vi "fifoTesting.vi"   [LabVIEW 2016]
uses:
  <vilib>/Platform/TimedLoop/XDataNode/timing_clust.ctl
  <vilib>/Platform/TimedLoop/XDataNode/nitl_modes.ctl
  <vilib>/Platform/TimedLoop/XDataNode/wakeup.ctl
  <vilib>/rvi/Emulation/niFpgaSctlEmulationGetInTimedLoop.vi
  <vilib>/rvi/Emulation/niFpgaEmulationReportErrorSimple.vi
  <vilib>/rvi/Emulation/niFpgaGetClockAttributes.vi
  <vilib>/rvi/Emulation/niFpgaCriticalErrorInLSC.vi
  <vilib>/rvi/interface/RandomDataEmulation/niFpgaRandomDataHandleErrors.vi
  <vilib>/platform/TimedLoop/XDataNode/XDataNode.xnode
  <vilib>/rvi/DataTransferAndStorage/Container/XNode/niFpgaContainer.xnode
  <vilib>/rvi/interface/RandomDataEmulation/nirviRandomDataFpgaReadWriteTemplate.vi
  <vilib>/Platform/TimedLoop/XDataNode/XDNodeRunTimeDep.lvlib
types:
  T1 = typedef "XDNodeRunTimeDep.lvlib/timing_clust.ctl" = cluster{"Expected End [f-1]":u64, "Actual End [f-1]":u64, "Finished Late? [f-1]":bool, "Expected End [i-1]":u64, "Actual End [i-1]":u64, "Finished Late? [i-1]":bool, "Expected Start [i]":u64, "Actual Start [i]":u64, "Expected Start [f]":u64, "Actual Start [f]":u64, "Source Name":string, "Structure Name":string, "Period":i64, "Deadline":i64, "Offset":i64, "Start":i64, "Priority":i32, "Timeout":i32, "Mode":T2, "Wakeup Reason":T3, "Error":errorcluster, "Source Type":string, "Secondary Source Type":string, "Global End Time":u64, "Global Start Time":u64, "Frame Duration":u64, "Iteration Duration":u64, "Assigned CPU":i32, "I/O Scan Engine Mode":u32}
  T2 = typedef "XDNodeRunTimeDep.lvlib/nitl_modes.ctl" = enum32{"No Change", "Process missed periods, maintain original phase", "Discard missed periods, maintain original phase", "Process missed periods, ignore original phase", "Discard missed periods, ignore original phase"}
  T3 = typedef "XDNodeRunTimeDep.lvlib/wakeup.ctl" = enum32{"Normal", "Aborted", "Asynchronous wakeup", "Timing source error", "Timed loop error", "Timeout"}
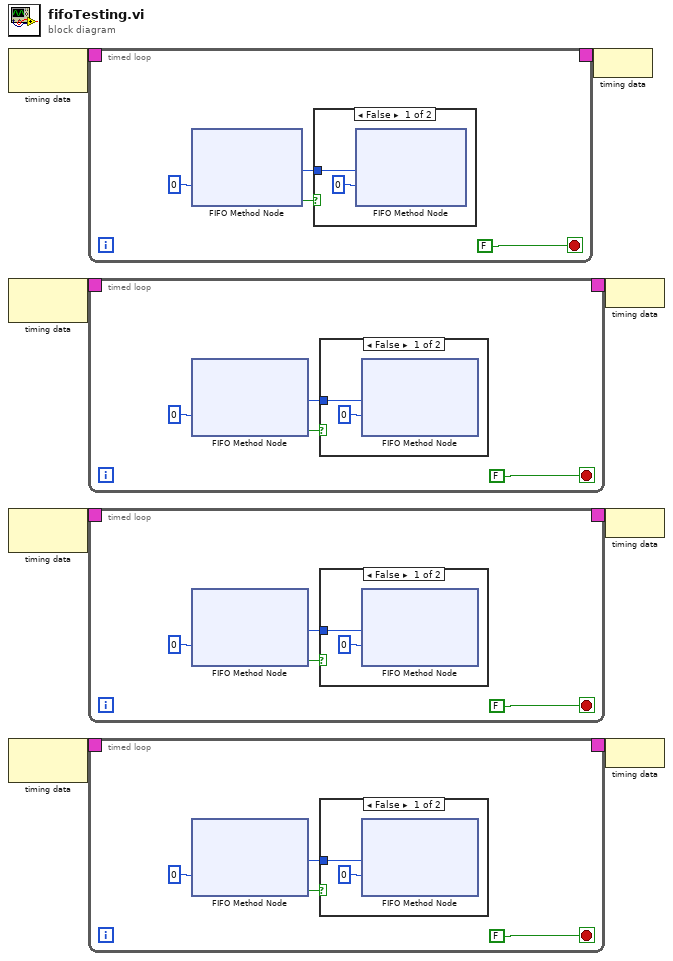
[diagram p0: block diagram]
diagram:
  n1 = node-c288() -> (w8:T1)  [unwired: 1 in]
  n2 = node-c288() -> (w6:T1)  [unwired: 1 in]
  n3 = node-c288() -> (w4:T1)  [unwired: 1 in]
  n4 = node-c288() -> (w2:T1)  [unwired: 1 in]
  n5 = timed-loop {
    timing: w8 -> [_]
    timing-out: [_] -> w7
    stop <- FALSE stop-if-true
    n6 = xnode ("FIFO Method Node")("Timeout"=0) -> ("Element"=w9:u8, "Timed Out?"=w10:bool)  [unwired: 1 in, 1 out]
    n7 = case shown="False" w10 {
      tunnel: w9 -> [w14 _]
      frame False {
        n8 = xnode ("FIFO Method Node")("Element"=w14, "Timeout"=0) -> ()  [unwired: 1 in, 2 out]
      }
      frame True {
      }
    }
  }
  n9 = timed-loop {
    timing: w6 -> [_]
    timing-out: [_] -> w5
    stop <- FALSE stop-if-true
    n10 = xnode ("FIFO Method Node")("Timeout"=0) -> ("Element"=w20:u16, "Timed Out?"=w19:bool)  [unwired: 1 in, 1 out]
    n11 = case shown="False" w19 {
      tunnel: w20 -> [w22 _]
      frame False {
        n12 = xnode ("FIFO Method Node")("Element"=w22, "Timeout"=0) -> ()  [unwired: 1 in, 2 out]
      }
      frame True {
      }
    }
  }
  n13 = timed-loop {
    timing: w4 -> [_]
    timing-out: [_] -> w3
    stop <- FALSE stop-if-true
    n14 = xnode ("FIFO Method Node")("Timeout"=0) -> ("Element"=w26:u32, "Timed Out?"=w27:bool)  [unwired: 1 in, 1 out]
    n15 = case shown="False" w27 {
      tunnel: w26 -> [w30 _]
      frame False {
        n16 = xnode ("FIFO Method Node")("Element"=w30, "Timeout"=0) -> ()  [unwired: 1 in, 2 out]
      }
      frame True {
      }
    }
  }
  n17 = timed-loop {
    timing: w2 -> [_]
    timing-out: [_] -> w1
    stop <- FALSE stop-if-true
    n18 = xnode ("FIFO Method Node")("Timeout"=0) -> ("Element"=w36:u64, "Timed Out?"=w35:bool)  [unwired: 1 in, 1 out]
    n19 = case shown="False" w35 {
      tunnel: w36 -> [w38 _]
      frame False {
        n20 = xnode ("FIFO Method Node")("Element"=w38, "Timeout"=0) -> ()  [unwired: 1 in, 2 out]
      }
      frame True {
      }
    }
  }
  n21 = node-c288(w7) -> ()
  n22 = node-c288(w5) -> ()
  n23 = node-c288(w3) -> ()
  n24 = node-c288(w1) -> ()
